vi "Set FPGA Reference.vi"(8 "Error In":errorcluster, 10 "FPGA VI Reference":T1, 11 "Display In":refnum<class "Display.lvclass">) -> (0 "Error Out":errorcluster, 3 "Display Out":refnum<class "Display.lvclass">)   [LabVIEW 2019, in "Display.lvclass"]
uses:
  Display.lvclass
  Public/Controls/FPGA Reference.ctl
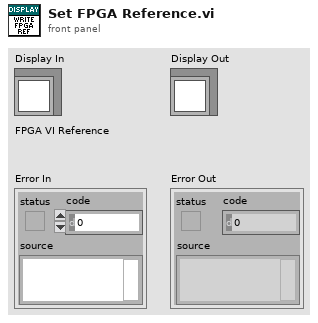
[diagram p1: front panel]
types:
  T1 = typedef "Display.lvclass/FPGA Reference.ctl" = refnum<k20>
  T2 = typedef "Display.lvclass/Data.ctl" = cluster{"Size":T3, "Display Elements":refnum<class "Display Element.lvclass">[], "Frame":u32[][], "RGB Gains":T4, "FPGA VI Reference":T1}
  T3 = typedef "Display Utilities.lvlib/2D Dimensions.ctl" = cluster{"Width":i32, "Height":i32}
  T4 = typedef "Display.lvclass/RGB Gains.ctl" = cluster{"Red":sgl, "Green":sgl, "Blue":sgl}
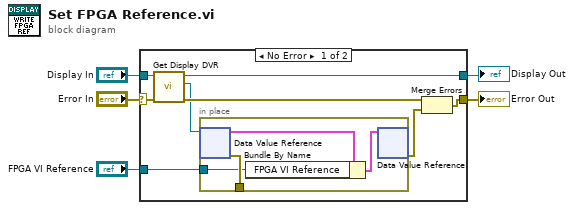
[diagram p0: block diagram]
diagram:
  n1 = case shown="No Error" "Error In" {
    selector: "Error In" -> [w10 w18]
    tunnel: [w12 w18] -> w1
    tunnel: [w7 w19] -> w2
    tunnel: "Display In" -> [w9 w19]
    tunnel: "FPGA VI Reference" -> [w11 _]
    frame No Error {
      n2 = call "Get Display DVR.vi"("Error In"=w10, "Display In"=w9) -> ("Error Out"=w8:errorcluster, "DVR"=w6:refnum<data-value>, "Display Out"=w7:refnum<class "Display.lvclass">)  [unwired: 7 in]
      n3 = in-place {
        in-place-border: [w17] -> _
        in-place-border: w11 -> [w14]
        n4 = in-place-dvr #1(w6) -> (w16:T2, w17:errorcluster)
        n5 = Bundle By Name(cluster=w16, "FPGA VI Reference"=w14) -> (w15:T2)
        n6 = in-place-dvr #1(w15) -> (w13:errorcluster)  [unwired: 1 out]
      }
      n7 = Merge Errors(w8, w13) -> (w12:errorcluster)
    }
    frame Error {
    }
  }
  "Error Out" <- w1
  "Display Out" <- w2
